vi "DroneFrontPanel.vi"() -> ()   [LabVIEW 2023]
doc: "Demonstrates how to open a connection to an TCP server, read the data being sent, and display the data on a chart. This VI is designed to stop if the TCP connection is terminated."
panel:
  out "String":string
  out "length 2":i32
  out "length":i32
  out "bytes written - opstijgen":i32
  out "bytes written":i32
  out "?":i32(slide) scale=0.0..100.0
  in  "Land":bool
  in  "Next Target":bool
  in  "Track":bool
  in  "?":bool
  in  "Rise":bool
  out "Webcam":picture
  in  "Server Closed":string="The server VI closed the connection."
  # "Overview: Demonstrates the use of the TCP functions to connect to a TCP server VI and receive data.\nInstructions:\n1. Ensure Simple TCP - Server.vi is already running.\n2. Run the VI.\n3. Click Stop to stop the VI. Note that if you stop the server VI, this VI will stop automatically."
  # "Following target"
  # "9/19/2023  22:04:26"
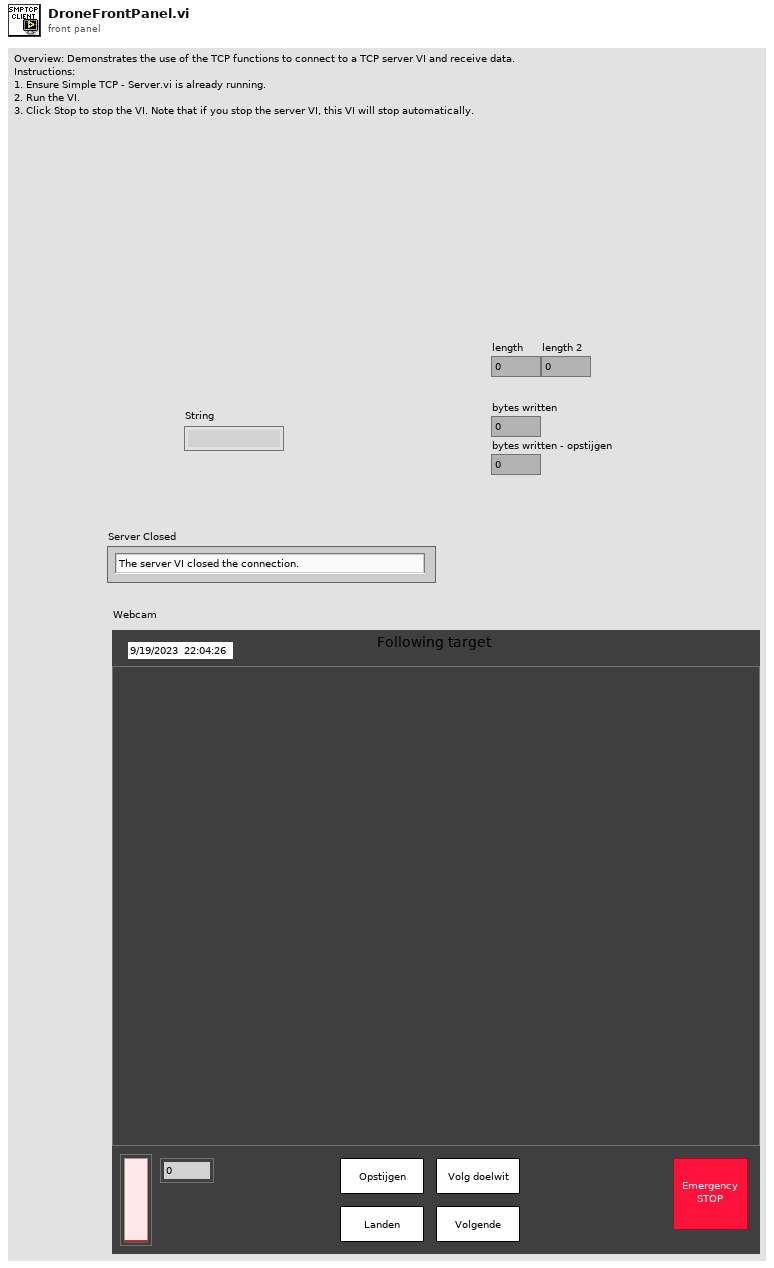
[diagram p1: front panel]
types:
  T1 = enum16{"Standard", "Buffered", "CRLF", "Immediate"}
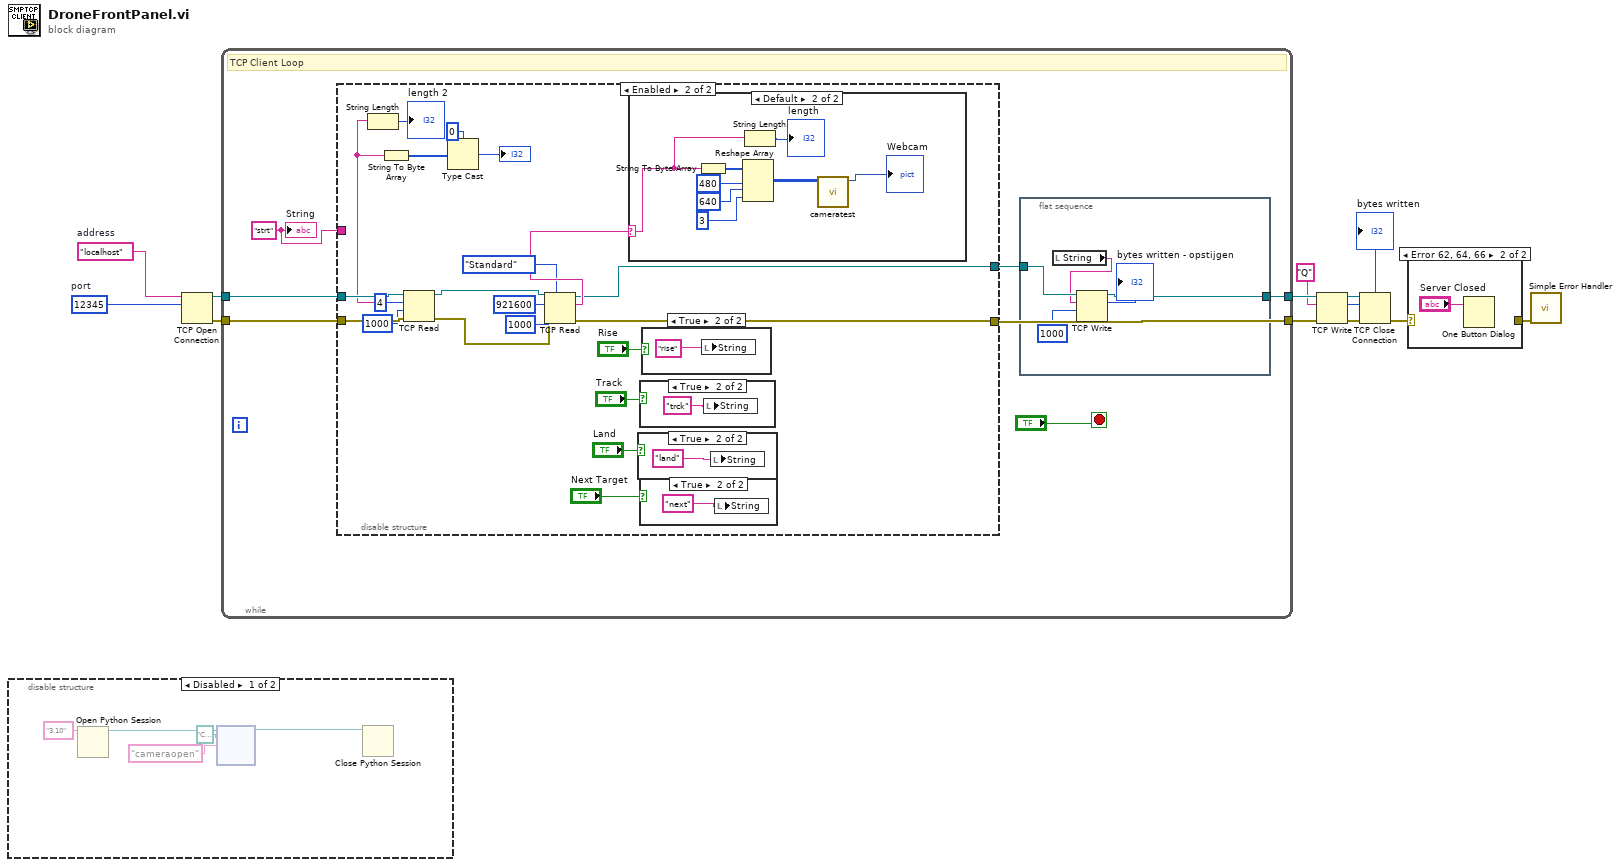
[diagram p0: block diagram]
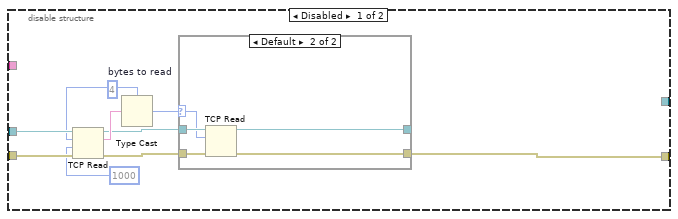
[diagram p4: hidden frame]
diagram:
  w2 = u16 12345  # port
  w3 = "localhost"  # address
  n1 = disable-structure shown="Disabled" {
    frame Disabled {
      n2 = Open Python Session(python version="3.10" ("Python version")) -> (session out=w16:refnum<k35>)  [unwired: 2 in, 1 out]
      n3 = node(w16, path "C:/Users/User/source/repos/PythonCameraTest/PythonCameraTest/tcpservertest.py" ("module path"), "cameraopen" ("function name")) -> (w15:refnum<k35>)  [unwired: 3 in, 3 out]
      n4 = Close Python Session(session in=w15) -> ()  [unwired: 1 in, 1 out]
    }
    frame Enabled {
    }
  }
  n5 = TCP Open Connection(address=w3, remote port or service name=w2) -> (connection ID=w12:refnum<k5>, error out=w11:errorcluster)  [unwired: 3 in]
  n6 = while {
    tunnel: w11 -> [w23]
    tunnel: w12 -> [w24]
    tunnel: [w18] -> w9
    tunnel: [w22] -> w7
    stop <- "?" stop-if-true
    w20 = "strt" ("String")
    # "TCP Client Loop"
    n7 = disable-structure shown="Enabled" {
      disable-tunnel: w24 -> [w36 w62]
      disable-tunnel: w23 -> [w35 w61]
      disable-tunnel: [w32 w50] -> w22
      disable-tunnel: w20 -> [_ _]
      disable-tunnel: [_ w51] -> w19
      frame Disabled {
        w34 = 4  # bytes to read
        n8 = TCP Read(connection ID=w36, bytes to read=w34, error in (no error)=w35, 9:1000 ("timeout ms (25000)")) -> (connection ID out=w38:refnum<k5>, data out=w39:string, error out=w37:errorcluster)  [unwired: 1 in]
        n9 = Type Cast(type=w34, x=w39) -> (*(type *) &x=w31:i32)
        n10 = case shown="Default" w31 {
          selector: w31 -> [_ w42]
          tunnel: w38 -> [w41 w46]
          tunnel: w37 -> [w40 w45]
          tunnel: [w41 w44] -> w33
          tunnel: [w40 w43] -> w32
          frame ..0 {
            # "The server has not written any data"
          }
          frame Default {
            n11 = TCP Read(connection ID=w46, bytes to read=w42, error in (no error)=w45) -> (connection ID out=w44:refnum<k5>, error out=w43:errorcluster)  [unwired: 2 in, 1 out]
          }
        }
      }
      frame Enabled {
        n12 = TCP Read(connection ID=w62, bytes to read=4, error in (no error)=w61, 9:1000 ("timeout ms (25000)")) -> (connection ID out=w59:refnum<k5>, data out=w55:string, error out=w58:errorcluster)  [unwired: 1 in]
        n13 = String Length(string=w55) -> (length=→"length 2":i32)
        n14 = String To Byte Array(string=w55) -> (unsigned byte array=w54:u8[])
        n15 = Type Cast(type=0, x=w54) -> (*(type *) &x=→"?":i32)
        n16 = TCP Read(connection ID=w59, bytes to read=921600, error in (no error)=w58, 7:T1."Standard" ("mode (standard)"), 9:1000 ("timeout ms (25000)")) -> (connection ID out=w51:refnum<k5>, data out=w67:string, error out=w50:errorcluster)
        n17 = case shown="Default" w67 {
          selector: w67 -> [_ w73]
          frame "" {
          }
          frame Default {
            n18 = String To Byte Array(string=w73) -> (unsigned byte array=w79:u8[])
            n19 = Reshape Array(w79, 480 ("dimension size"), 640 ("dimension size"), 3 ("dimension size")) -> (w75:u8[][][])
            n20 = String Length(string=w73) -> (length=→"length":i32)
            n21 = call "cameratest.vi"("return value"=w75) -> ("Webcam footage"=→"Webcam":picture)  [unwired: 10 in]
          }
        }
        n22 = case shown="True" "Land" {
          frame False {
          }
          frame True {
            n23 = local write "String"("land" ("String")) -> ()
          }
        }
        n24 = case shown="True" "Track" {
          frame False {
          }
          frame True {
            n25 = local write "String"("trck" ("String")) -> ()
          }
        }
        n26 = case shown="True" "Next Target" {
          frame False {
          }
          frame True {
            n27 = local write "String"("next" ("String")) -> ()
          }
        }
        n28 = case shown="True" "Rise" {
          frame False {
          }
          frame True {
            n29 = local write "String"("rise" ("data in")) -> ()
          }
        }
      }
    }
    n30 = flat-sequence {
      tunnel: w19 -> [w27]
      tunnel: [w26] -> w18
      frame #0 {
        n31 = local read "String"() -> (w25:string)
        n32 = TCP Write(connection ID=w27, data in=w25, 9:1000 ("timeout ms (25000)")) -> (connection ID out=w26:refnum<k5>, bytes written=→"bytes written - opstijgen":i32)  [unwired: 1 in, 1 out]
      }
    }
    "String" <- w20
  }
  n33 = TCP Write(connection ID=w9, data in="Q", error in (no error)=w7) -> (connection ID out=w10:refnum<k5>, bytes written=→"bytes written":i32, error out=w8:errorcluster)  [unwired: 1 out]
  n34 = TCP Close Connection(connection ID=w10, error in (no error)=w8) -> (error out=w5:errorcluster)  [unwired: 1 in, 1 out]
  n35 = case shown="Error 62, 64, 66" w5 {
    selector: w5 -> [w80 _]
    tunnel: [w80 _] -> w4
    frame #0 {
    }
    frame #1 {
      n36 = One Button Dialog(message="Server Closed") -> ()  [unwired: 1 in, 1 out]
    }
  }
  n37 = call <vilib>:"Simple Error Handler.vi"("error in (no error)"=w4) -> ()  [unwired: 4 in, 5 out]
